vi "Set Control Value by Name.vi"(8 "Control Data (Variant)":variant, 9 "Control Label":string, 10 "error in":errorcluster, 11 "VI  Ref":refnum<vi>) -> (2 "error out":errorcluster, 3 "VI  Ref (out)":refnum<vi>)   [LabVIEW 2021, in "Utilities.lvlib"]
doc: "Returns an array of control refnums, labels and data, from the front panel of the calling VI.\n\nThis VI also accounts for tab controls within other tab controls."
uses:
  Utilities.lvlib
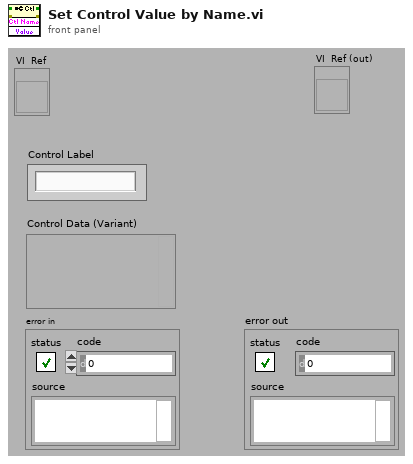
[diagram p1: front panel]
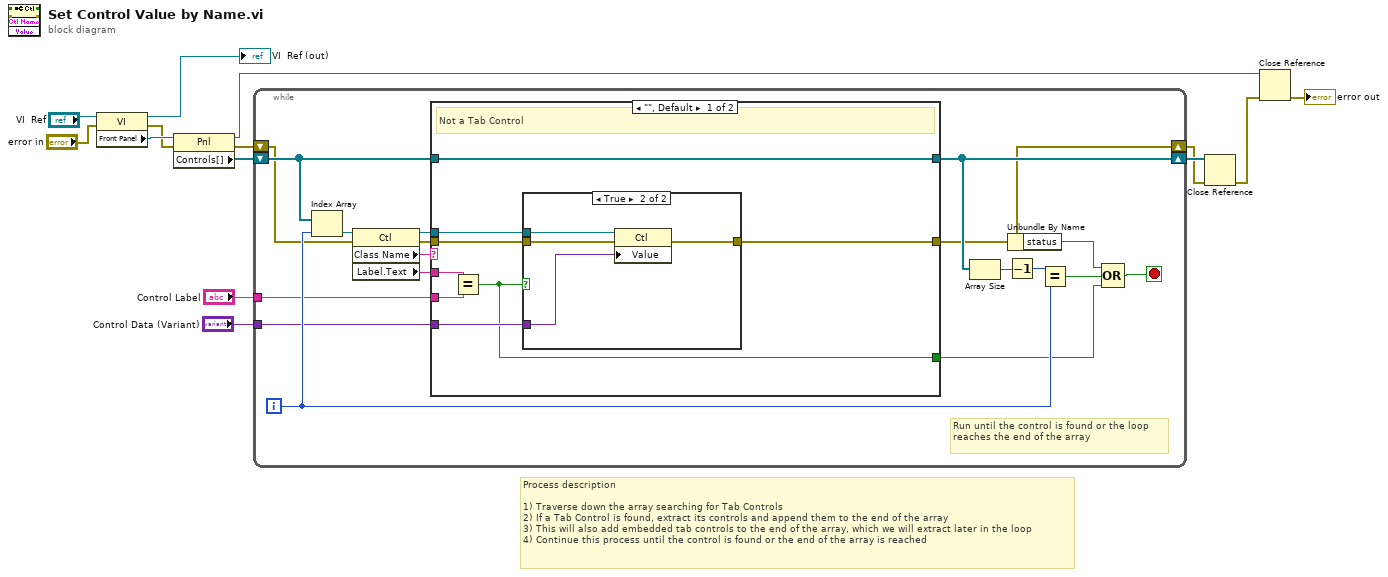
[diagram p0: block diagram]
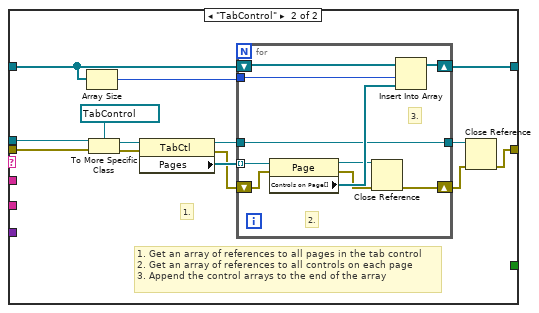
[diagram p3: hidden frame]
diagram:
  # "Process description\n\n1) Traverse down the array searching for Tab Controls\n2) If a Tab Control is found, extract its controls and append them to the end of the array\n3) This will also add embedded tab controls to the end of the array, which we will extract later in the loop\n4) Continue this process until the control is found or the end of the array is reached"
  n1 = property class="VI"(reference="VI  Ref", error in="error in") -> (reference out=→"VI  Ref (out)":refnum<vi>, error out=w12:errorcluster, "Front Panel"=w13:refnum<vi>)
  n2 = property class="Pnl"(reference=w13, error in=w12) -> (reference out=w10:refnum<vi>, error out=w11:errorcluster, "Controls[]"=w14:refnum<vi>[])
  n3 = while {
    shift-right: [w25] -> w3
    shift-left: w14 -> [w31]
    shift-right: [w22] -> w2
    shift-left: w11 -> [w24]
    tunnel: "Control Label" -> [w17]
    tunnel: "Control Data (Variant)" -> [w16]
    i -> [w26]
    stop <- w20 stop-if-true
    # "Run until the control is found or the loop reaches the end of the array"
    n4 = Index Array(array=w31, index=w26) -> (element=w27:refnum<vi>)
    n5 = property class="Ctl"(reference=w27, error in=w24) -> (reference out=w32:refnum<vi>, error out=w23:errorcluster, "Class Name"=w30:string, "Label.Text"=w18:string)
    n6 = case shown="\"\", Default" w30 {
      tunnel: w32 -> [w35 w59]
      tunnel: w31 -> [w40 w55]
      tunnel: [w40 w56] -> w25
      tunnel: w23 -> [w37 w52]
      tunnel: [w36 w48] -> w22
      tunnel: w18 -> [w39 _]
      tunnel: w17 -> [w38 _]
      tunnel: w16 -> [w34 _]
      tunnel: [w33 _] -> w15
      frame "", Default {
        # "Not a Tab Control"
        n7 = Equal?(x=w39, y=w38) -> (x = y?=w33:bool)
        n8 = case shown="True" w33 {
          tunnel: w37 -> [w41 w45]
          tunnel: [w41 w44] -> w36
          tunnel: w35 -> [_ w43]
          tunnel: w34 -> [_ w42]
          frame False {
          }
          frame True {
            n9 = property class="Ctl"(reference=w43, error in=w45, "Value"=w42) -> (error out=w44:errorcluster)  [unwired: 1 out]
          }
        }
      }
      frame "TabControl" {
        # "1. Get an array of references to all pages in the tab control\n2. Get an array of references to all controls on each page\n3. Append the control arrays to the end of the array"
        # "1."
        n10 = Array Size(array=w55) -> (size(s)=w53:i32)
        n11 = To More Specific Class(target class=refnum<vi> refnum ("Tab Control"), reference=w59, error in=w52) -> (specific class reference=w58:refnum<vi>, error out=w51:errorcluster)
        n12 = property class="TabCtl"(reference=w58, error in=w51) -> (reference out=w49:refnum<vi>, error out=w50:errorcluster, "Pages"=w57:refnum<vi>[])
        n13 = for {
          tunnel: w57 -> [w69] mode=indexing
          tunnel: w53 -> [w67]
          shift-right: [w68] -> w56
          shift-left: w55 -> [w66]
          tunnel: w49 -> [w63]
          tunnel: [w63] -> w47
          shift-right: [w60] -> w46
          shift-left: w50 -> [w64]
          # "3."
          # "2."
          n14 = property class="Page"(reference=w69, error in=w64) -> (reference out=w62:refnum<vi>, error out=w61:errorcluster, "Controls on Page[]"=w65:refnum<vi>[])
          n15 = Close Reference(reference=w62, error in (no error)=w61) -> (error out=w60:errorcluster)
          n16 = Insert Into Array(array=w66, index=w67, new element=w65) -> (w68:refnum<vi>[])
        }
        n17 = Close Reference(reference=w47, error in (no error)=w46) -> (error out=w48:errorcluster)
      }
    }
    n18 = Array Size(array=w25) -> (size(s)=w29:i32)
    n19 = Decrement(x=w29) -> (x-1=w28:i32)
    n20 = Unbundle By Name(w22) -> ("status"=w19:bool)
    n21 = Equal?(x=w28, y=w26) -> (x = y?=w21:bool)
    n22 = Compound Arithmetic op=OR(w19, w21, w15) -> (w20:bool)
  }
  n23 = Close Reference(reference=w3, error in (no error)=w2) -> (error out=w1:errorcluster)
  n24 = Close Reference(reference=w10, error in (no error)=w1) -> (error out=→"error out":errorcluster)
